vi "ReadTriggered.vi"(8 "error in (no error)":errorcluster, 10 "Keep last record only":bool, 11 "Scope5761 in":refnum<class "Scope5761.lvclass">) -> (0 "error out":errorcluster, 1 "#elements":i32, 2 "Data":dbl[][](array[numeric]), 3 "Scope5761 out":refnum<class "Scope5761.lvclass">)   [LabVIEW 2013, in "Scope5761.lvclass"]
uses:
  Scope5761.lvclass
  Scope5761.lvclass/Scope5761.ctl
  FpgaRef/FpgaRef5761/FpgaRef5761.lvclass
  FpgaRef/FpgaRef5782/FpgaRef5782.lvclass
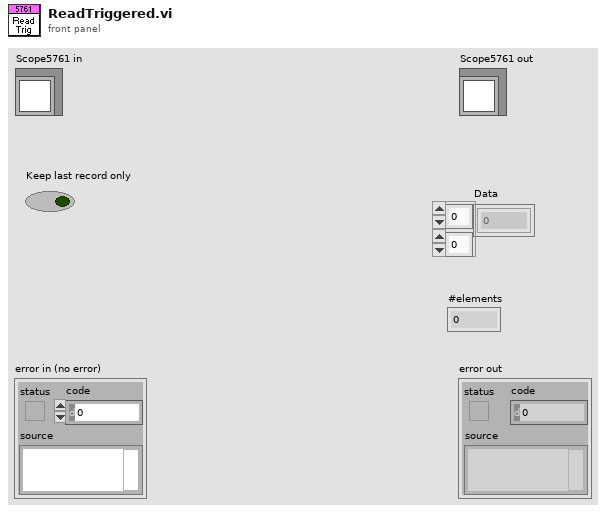
[diagram p1: front panel]
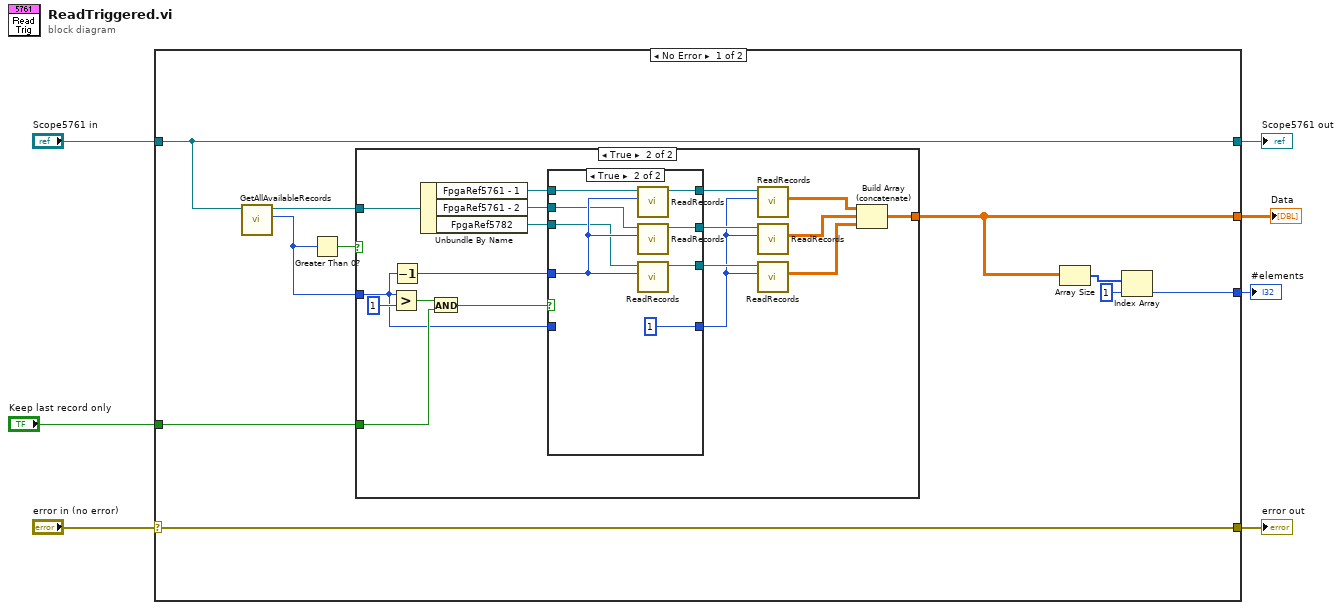
[diagram p0: block diagram]
diagram:
  n1 = case shown="No Error" "error in (no error)" {
    selector: "error in (no error)" -> [w17 w49]
    tunnel: [w17 w49] -> w6
    tunnel: [w16 w48] -> w4
    tunnel: "Scope5761 in" -> [w16 w48]
    tunnel: "Keep last record only" -> [w13 _]
    tunnel: [w11 _] -> w2
    tunnel: [w8 _] -> w1
    frame No Error {
      n2 = call-dynamic "GetAllAvailableRecords.vi"("Scope5761 in"=w16) -> ("Available records"=w12:i32, "Scope5761 out"=w14:refnum<class "Scope5761.lvclass">)  [unwired: 8 in, 1 out]
      n3 = Greater Than 0?(x=w12) -> (x > 0?=w15:bool)
      n4 = case shown="True" w15 {
        tunnel: w14 -> [_ w30]
        tunnel: w13 -> [_ w33]
        tunnel: w12 -> [_ w26]
        tunnel: [_ w18] -> w11
        frame False {
        }
        frame True {
          n5 = Greater?(x=w26, y=1) -> (0:w34:bool)
          n6 = Decrement(x=w26) -> (x-1=w31:i32)
          n7 = Unbundle By Name(w30) -> ("FpgaRef5761 - 1"=w29:refnum<class "FpgaRef5761.lvclass">, "FpgaRef5761 - 2"=w28:refnum<class "FpgaRef5761.lvclass">, "FpgaRef5782"=w27:refnum<class "FpgaRef5782.lvclass">)
          n8 = And(x=w34, y=w33) -> (x .and. y?=w32:bool)
          n9 = case shown="True" w32 {
            tunnel: w31 -> [_ w47]
            tunnel: w29 -> [w38 w46]
            tunnel: w28 -> [w37 w45]
            tunnel: w27 -> [w36 w44]
            tunnel: [w38 w43] -> w25
            tunnel: [w37 w42] -> w24
            tunnel: [w36 w41] -> w23
            tunnel: [w39 1 ("y")] -> w22
            tunnel: w26 -> [w39 _]
            frame False {
            }
            frame True {
              n10 = call-dynamic "ReadRecords.vi"("Num records to read"=w47, "FpgaRef5761 In"=w46) -> ("FpgaRef5761 Out"=w43:refnum<class "FpgaRef5761.lvclass">)  [unwired: 7 in, 2 out]
              n11 = call-dynamic "ReadRecords.vi"("Num records to read"=w47, "FpgaRef5761 In"=w45) -> ("FpgaRef5761 Out"=w42:refnum<class "FpgaRef5761.lvclass">)  [unwired: 7 in, 2 out]
              n12 = call-dynamic "ReadRecords.vi"("Num records to read"=w47, "FpgaRef5782 in"=w44) -> ("FpgaRef5782 out"=w41:refnum<class "FpgaRef5782.lvclass">)  [unwired: 7 in, 2 out]
            }
          }
          n13 = call-dynamic "ReadRecords.vi"("Num records to read"=w22, "FpgaRef5761 In"=w25) -> ("Data"=w21:dbl[][])  [unwired: 7 in, 2 out]
          n14 = call-dynamic "ReadRecords.vi"("Num records to read"=w22, "FpgaRef5761 In"=w24) -> ("Data"=w20:dbl[][])  [unwired: 7 in, 2 out]
          n15 = call-dynamic "ReadRecords.vi"("Num records to read"=w22, "FpgaRef5782 in"=w23) -> ("Data"=w19:dbl[][])  [unwired: 7 in, 2 out]
          n16 = Build Array (concatenate)(w21, w20, w19) -> (w18:dbl[][])
        }
      }
      n17 = Array Size(array=w11) -> (size(s)=w10:i32[])
      n18 = Index Array(array=w10, index=1) -> (element=w8:i32)
    }
    frame Error {
    }
  }
  "error out" <- w6
  "Scope5761 out" <- w4
  "Data" <- w2
  "#elements" <- w1
